vi "Custom_Message.vi"(0 "Title":string, 5 "Message":string, 6 "OK Button":bool, 11 "Error_In":errorcluster, 13 "Path_Visible (F)":bool) -> (4 "Path_Out":path, 15 "Error_Out":errorcluster)   [LabVIEW 2021]
doc: "Its a custom message popup vi to prompt the user."
panel:
  in  "Path_In":path
  out "Messag_Out":string
  out "Title_Out":string
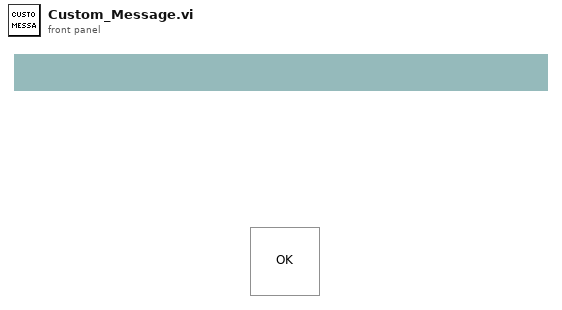
[diagram p1: front panel]
types:
  T1 = enum32{"Invalid", "Standard", "Closed", "Hidden", "Minimized", "Maximized"}
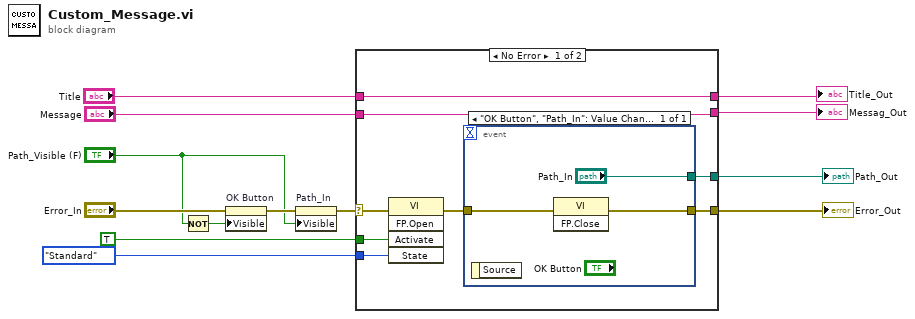
[diagram p0: block diagram]
diagram:
  n1 = Not(x="Path_Visible (F)") -> (.not. x?=w8:bool)
  n2 = property on="OK Button" class="Bool (strict)"(error in="Error_In", "Visible"=w8) -> (error out=w11:errorcluster)  [unwired: 1 in, 1 out]
  n3 = property on="Path_In" class="Path"(error in=w11, "Visible"="Path_Visible (F)") -> (error out=w9:errorcluster)  [unwired: 1 in, 1 out]
  n4 = case shown="No Error" w9 {
    selector: w9 -> [w21 w25]
    tunnel: [w17 w25] -> w1
    tunnel: TRUE ("Activate?") -> [w20 _]
    tunnel: T1."Standard" ("State") -> [w19 _]
    tunnel: [w18 _] -> w7
    tunnel: "Title" -> [w16 _]
    tunnel: [w16 _] -> w5
    tunnel: [w15 _] -> w4
    tunnel: "Message" -> [w15 _]
    frame No Error {
      n5 = invoke class="VI" method="FP.Open"(error in=w21, "Activate"=w20, "State"=w19) -> (error out=w14:errorcluster)  [unwired: 2 in, 4 out]
      n6 = event shown="[0] \"OK Button\", \"Path_In\": Value Change" {
        selector: _ -> [_]
        dyn-events: _ -> [_]
        timeout: _ -> [_]
        tunnel: [w24] -> w17
        tunnel: ["Path_In"] -> w18
        tunnel: w14 -> [w22]
        event "OK Button", "Path_In": Value Change {
          n7 = event-data() -> ()  [unwired: 1 in, 1 out]
          n8 = invoke class="VI" method="FP.Close"(error in=w22) -> (error out=w24:errorcluster)  [unwired: 2 in, 2 out]
        }
      }
    }
    frame Error {
    }
  }
  "Error_Out" <- w1
  "Path_Out" <- w7
  "Title_Out" <- w5
  "Messag_Out" <- w4
